vi "reset_timeout.vi"(8 "error in (no error)":errorcluster, 11 "ExperimentVariables in":refnum<class "ExperimentVariables.lvclass">) -> (0 "error out":errorcluster, 3 "ExperimentVariables out":refnum<class "ExperimentVariables.lvclass">)   [LabVIEW 2013, in "ExperimentVariables.lvclass"]
uses:
  ExperimentVariables.lvclass
  ExperimentVariables.lvclass/ExperimentVariables.ctl
  Experiment/Globals.vi
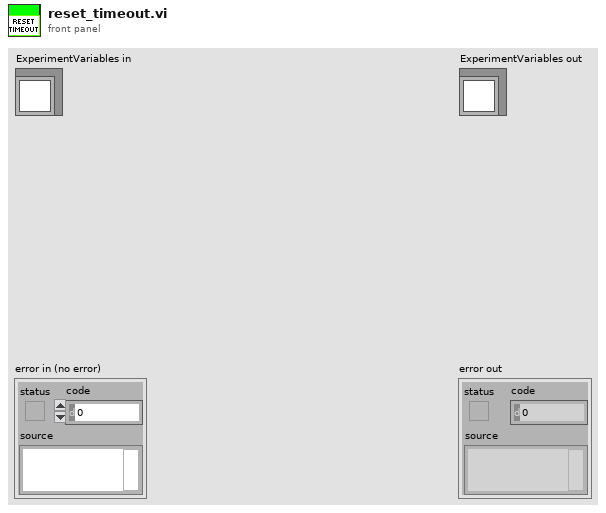
[diagram p1: front panel]
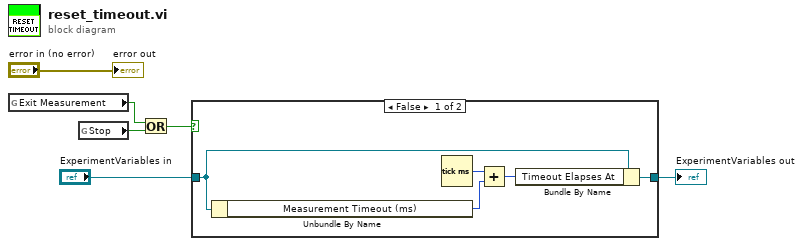
[diagram p0: block diagram]
diagram:
  n1 = global read "Globals.vi" "Exit Measurement"() -> (w3:bool)
  n2 = global read "Globals.vi" "Stop"() -> (w2:bool)
  n3 = Or(x=w3, y=w2) -> (x .or. y?=w1:bool)
  n4 = case shown="False" w1 {
    tunnel: [w11 w12] -> w5
    tunnel: "ExperimentVariables in" -> [w10 w12]
    frame False {
      n5 = Unbundle By Name(w10) -> ("Measurement Timeout (ms)"=w7:u32)
      n6 = Tick Count (ms)() -> (millisecond timer value=w9:u32)
      n7 = Add(x=w9, y=w7) -> (x+y=w8:u32)
      n8 = Bundle By Name(cluster=w10, "Timeout Elapses At"=w8) -> (w11:refnum<class "ExperimentVariables.lvclass">)
    }
    frame True {
    }
  }
  "ExperimentVariables out" <- w5
  "error out" <- "error in (no error)"
